vi "PID tank.vi"() -> ()   [LabVIEW 2020]
uses:
  <vilib>/addons/control/pid/pid.llb/PID Advanced (DBL).vi
  <vilib>/addons/control/pid/NI_PID_pid.lvlib
panel:
  in  "stop":bool
  in  "auto? (T)":bool=TRUE
  in  "Control Valve":dbl format="%.2f"
  in  "Process Parameters":T1={"static gain"=2.5, "lag (s)"=2.5, "deadtime (s)"=0.001, "load"=0.0, "deadband"=0.0, "sensor noise"=0.0, "initial PV"=30.0, "plant noise"=0.0} {"plant noise" format="%.2f"; "initial PV" format="%.2f"; "sensor noise" format="%.2f"; "lag (s)" format="%.2f"; "deadtime (s)" format="%.2f"; "deadband" format="%.1f"; "load" format="%.2f"; "static gain" format="%.2f"}
  in  "PID gains":T2={"proportional gain (Kc)"=1.0, "integral time (Ti, min)"=0.01, "derivative time (Td, min)"=0.0} {"derivative time (Td, min)" format="%.3f"; "integral time (Ti, min)" format="%.3f"; "proportional gain (Kc)" format="%.3f"}
  out "Control Valve":dbl(knob) scale=0.0..100.0
  out "Waveform Chart":T3(graph)
  in  "Set Point":dbl(slide) scale=0.0..100.0
  out "Process Variable":dbl(slide) scale=0.0..100.0
  # "IN"
  # "OUT"
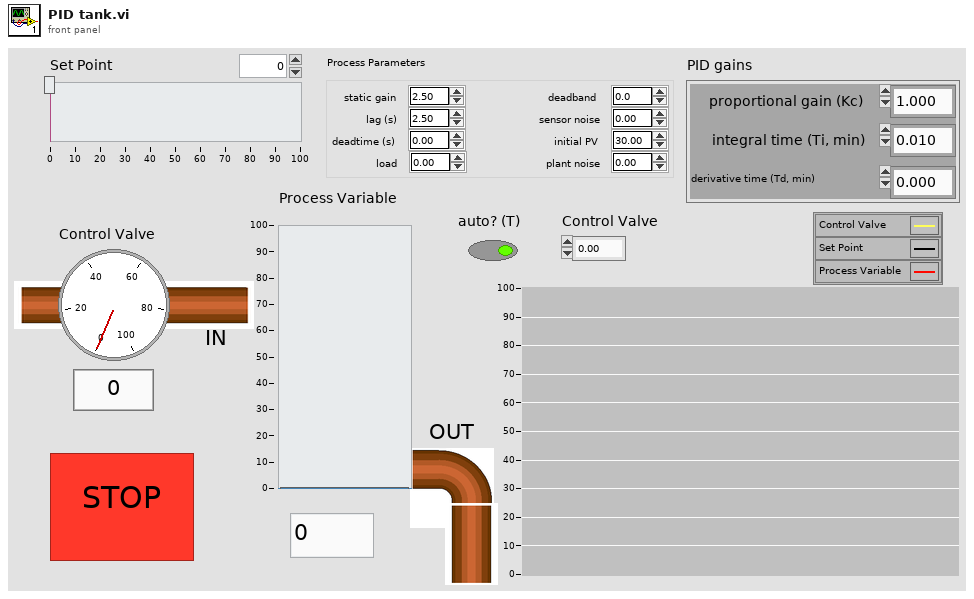
[diagram p1: front panel]
types:
  T1 = cluster{"static gain":dbl, "lag (s)":dbl, "deadtime (s)":dbl, "load":dbl, "deadband":dbl, "sensor noise":dbl, "initial PV":dbl, "plant noise":dbl}
  T2 = cluster{"proportional gain (Kc)":dbl, "integral time (Ti, min)":dbl, "derivative time (Td, min)":dbl}
  T3 = cluster{"output":dbl, "Set Point":dbl, "Plant Output":dbl}
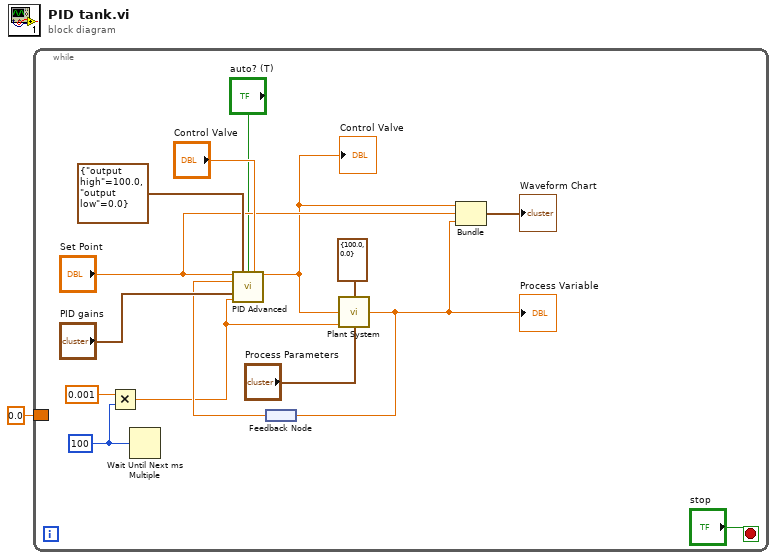
[diagram p0: block diagram]
diagram:
  n1 = while {
    border: 0.0 ("Plant Output") -> [_]
    stop <- "stop" stop-if-true
    w9 = u32 100 ("millisecond multiple")
    n2 = Multiply(x=0.001, y=w9) -> (x*y=w8:dbl)
    n3 = Wait Until Next ms Multiple(millisecond multiple=w9) -> ()  [unwired: 1 out]
    n4 = feedback #1() -> (w13:dbl)
    n5 = call-poly <vilib>:"PID Advanced.vi"("setpoint"="Set Point", "output range"=cluster{"output high":dbl, "output low":dbl} {"output high"=100.0, "output low"=0.0}, "auto? (T)"="auto? (T)", "manual control"="Control Valve", "process variable"=w13, "PID gains"="PID gains", "dt (s)"=w8) -> ("output"=w5:dbl)  [unwired: 7 in, 1 out]
    "Control Valve" <- w5
    n6 = call "Plant System.vi"("output saturation range"=cluster{"output high":dbl, "output low":dbl} {"output high"=100.0, "output low"=0.0}, "Plant Input"=w5, "dt (s)"=w8, "process parameters"="Process Parameters") -> ("Plant Output"=w7:dbl)  [unwired: 11 in]
    "Process Variable" <- w7
    n7 = feedback-in #1(w7) -> ()
    n8 = Bundle("output"=w5, "Set Point"="Set Point", "Plant Output"=w7) -> (→"Waveform Chart":T3)  [unwired: 1 in]
  }
